vi "RSZVB Set Marker Format.vi"(7 "Marker Format (0: dB Mag)":i32(ring) items=["dB Mag"=0, "Lin Mag"=6, "Phase"=1, "Real"=7, "Imag"=8, "SWR"=5, "Delay"=4, "dB Mag and Phase"=11, "Lin Mag and Phase"=12, "Real and Imag"=13, "Default (Trace)"=14, "R + j X"=15, "G + j B"=16], 8 "error in (no error)":errorcluster {"code" format="%.0x"}, 9 "Marker (1)":i32=1, 10 "Channel (Trace) (1)":i32=1, 11 "VISA session":refnum<visa-resource-name>) -> (0 "error out":errorcluster {"code" format="%.0x"}, 3 "dup VISA session":refnum<visa-resource-name>)   [LabVIEW 2011]
doc: "This VI defines the output format for the (complex) value of marker <Mk> on trace no. <Ch/Tr>.\n\nNote(s):\n\nThe formats of the markers assigned to a trace are independent of each other and of the trace format settings; see CALCulate<Ch/Tr>:FORMat.\n\nRemote-control command(s):\nCALCulate<Ch/Tr>:MARKer<Mk>:FORMat MLINear | MLOGarithmic | PHASe | POLar | COMPlex | GDELay | REAL | IMAGinary | SWR | LINPhase | LOGPhase | IMPedance | ADMittance | MDB | MLPHas | MDPHase"
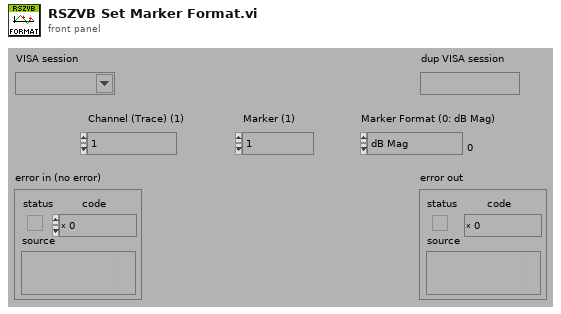
[diagram p1: front panel]
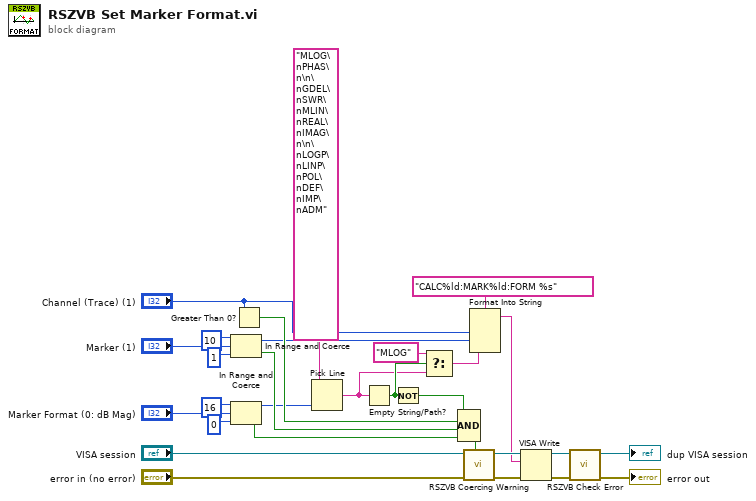
[diagram p0: block diagram]
diagram:
  n1 = In Range and Coerce(upper limit=10, x="Marker (1)", lower limit=1) -> (coerced(x)=w18:i32, In Range?=w19:bool)
  n2 = In Range and Coerce(upper limit=16, x="Marker Format (0: dB Mag)", lower limit=0) -> (coerced(x)=w13:i32, In Range?=w15:bool)
  n3 = Greater Than 0?(x="Channel (Trace) (1)") -> (x > 0?=w22:bool)
  n4 = Pick Line(multi-line string="MLOG\nPHAS\n\n\nGDEL\nSWR\nMLIN\nREAL\nIMAG\n\n\nLOGP\nLINP\nPOL\nDEF\nIMP\nADM", line index=w13) -> (output string=w2:string)  [unwired: 1 in]
  n5 = Empty String/Path?(string/path=w2) -> (empty?=w3:bool)
  n6 = Not(x=w3) -> (.not. x?=w5:bool)
  n7 = Select(t="MLOG", s=w3, f=w2) -> (s? t:f=w4:string)
  n8 = Compound Arithmetic op=AND(w5, w22, w19, w15) -> (w24:bool)
  n9 = call "RSZVB Coercing Warning.vi"("In Range?"=w24, "error in (no error)"="error in (no error)", "VISA session"="VISA session") -> ("error out"=w27:errorcluster, "dup VISA session"=w28:refnum<visa-resource-name>)  [unwired: 7 in]
  n10 = Format Into String(format string="CALC%ld:MARK%ld:FORM %s", "Channel (Trace) (1)", w18, w4) -> (resulting string=w23:string)  [unwired: 2 in, 1 out]
  n11 = VISA Write(VISA resource name=w28, write buffer=w23, error in (no error)=w27) -> (VISA resource name out=w25:refnum<visa-resource-name>, error out=w26:errorcluster)  [unwired: 1 out]
  n12 = call "RSZVB Check Error.vi"("error in (no error)"=w26, "VISA session"=w25) -> ("error out"=→"error out":errorcluster, "dup VISA session"=→"dup VISA session":refnum<visa-resource-name>)  [unwired: 8 in]
